vi "_DServerSetAttributeInfo.vi"(2 "error in":errorcluster, 3 "attribute info":T1) -> (0 "error out":errorcluster)   [LabVIEW 2014, in "tango.lvlib"]
uses:
  tango.lvlib
  tango_binding.so
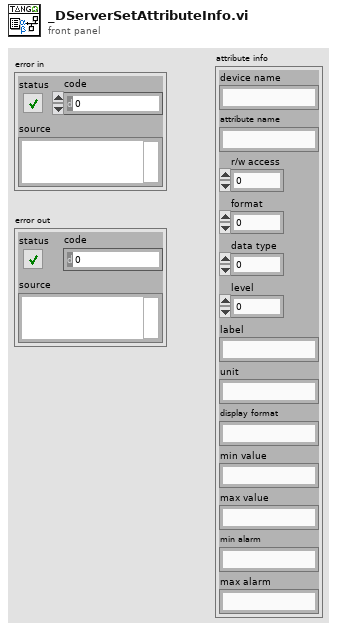
[diagram p1: front panel]
types:
  T1 = cluster{"device name":string, "attribute name":string, "r/w access":i16, "format":i16, "data type":i16, "level":i16, "label":string, "unit":string, "display format":string, "min value":string, "max value":string, "min alarm":string, "max alarm":string}
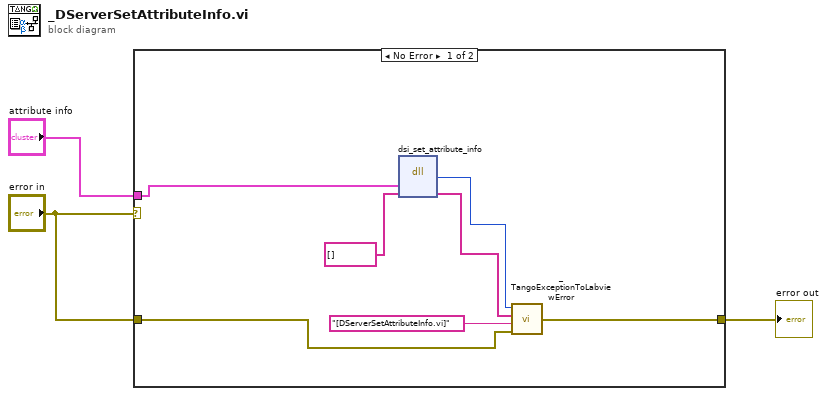
[diagram p0: block diagram]
diagram:
  n1 = case shown="No Error" "error in" {
    tunnel: [w9 w11] -> w2
    tunnel: "error in" -> [w8 w11]
    tunnel: "attribute info" -> [w4 _]
    frame No Error {
      n2 = dll-call lib="tango_binding.*" fn="dsi_set_attribute_info"("attrs_info_inout"=w4, "error_stack"=string[] [] ("error stack")) -> ("return type"=w5:i32, "error_stack"=w6:string[])  [unwired: 4 in, 2 out]
      n3 = call "_TangoExceptionToLabviewError.vi"("error in"=w8, "location"="[DServerSetAttributeInfo.vi]", "error stack"=w6, "error code"=w5) -> ("error out"=w9:errorcluster)
    }
    frame Error {
    }
  }
  "error out" <- w2
